vi "ping.vi"(8 "error in (no error)":errorcluster, 11 "stub in":refnum<class "stub.lvclass">) -> (0 "error out":errorcluster, 2 "Ping OK":bool, 3 "stub out":refnum<class "stub.lvclass">)   [LabVIEW 2021, in "stub.lvclass"]
uses:
  stub.lvclass
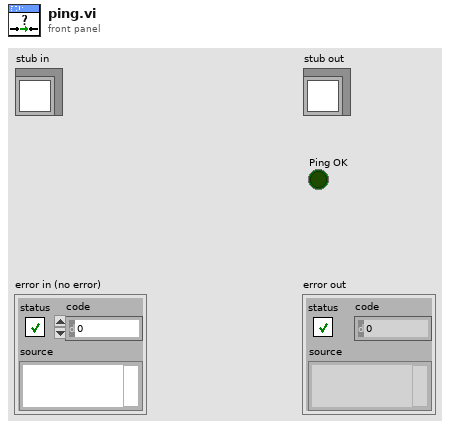
[diagram p1: front panel]
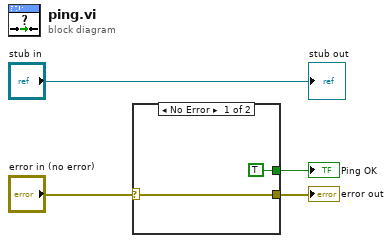
[diagram p0: block diagram]
diagram:
  n1 = case shown="No Error" "error in (no error)" {
    selector: "error in (no error)" -> [w5 w7]
    tunnel: [w5 w7] -> w3
    tunnel: [TRUE ("OK") _] -> w1
    frame No Error {
    }
    frame Error {
    }
  }
  "error out" <- w3
  "Ping OK" <- w1
  "stub out" <- "stub in"
